vi "Destructor.vi"(8 "error in (no error)":errorcluster, 11 "Collection in":refnum<class "CollectionByValue.lvclass">) -> (0 "error out":errorcluster)   [LabVIEW 2021, in "Collection.lvlib" / "CollectionByValue.lvclass"]
uses:
  CollectionByValue.lvclass
  CollectionByValue.lvclass/CollectionByValue.ctl
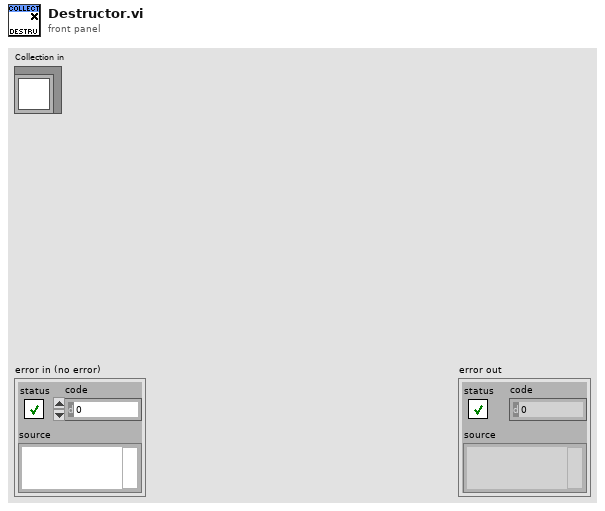
[diagram p1: front panel]
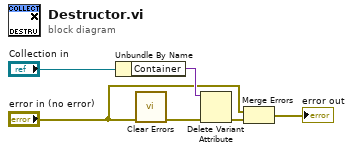
[diagram p0: block diagram]
diagram:
  n1 = Unbundle By Name("Collection in") -> ("Container"=w5:variant)
  n2 = call <vilib>:"Clear Errors.vi"("error in (no error)"="error in (no error)") -> ("error out"=w4:errorcluster)  [unwired: 5 in, 1 out]
  n3 = Delete Variant Attribute(4:w4, 7:w5) -> (0:w3:errorcluster)  [unwired: 1 in, 2 out]
  n4 = Merge Errors("error in (no error)", w3) -> (→"error out":errorcluster)
